vi "Set supply output on first loop.vi"(4 "Current":dbl=300.0 format="%#_gA", 6 "Voltage rise time":dbl=5.0 format="%#_13gs", 7 "Voltage":dbl=52.0 min=0.0 format="%.2fV", 9 "Numeric":i32, 10 "Power supply watchdog time":dbl=2.0 min=0.0 max=10.0 step=0.1 format="%#_13gs", 11 "VISA Refnum in":refnum<visa-resource-name>) -> (0 "error out":errorcluster, 3 "VISA Refnum out":refnum<visa-resource-name>)   [LabVIEW 2024]
uses:
  <userlib>/ZeroJet/IT6000C/IT6000C production.lvlib
  <instrlib>/IT6000C/IT6000C.lvlib
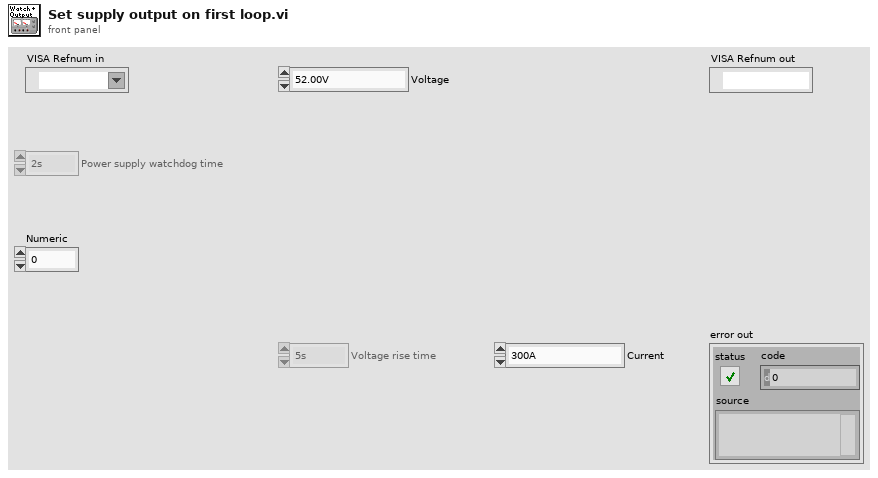
[diagram p1: front panel]
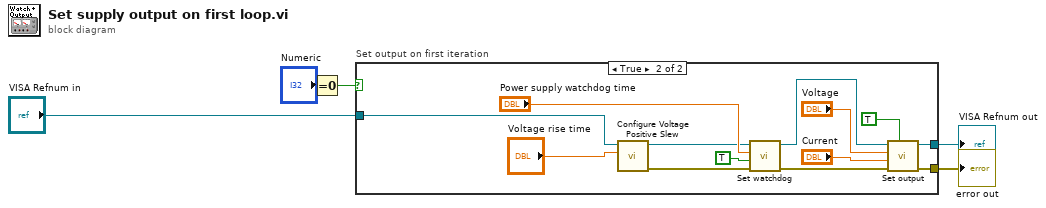
[diagram p0: block diagram]
diagram:
  n1 = Equal To 0?(x="Numeric") -> (x = 0?=w5:bool)
  n2 = case "Set output on first iteration" shown="True" w5 {
    tunnel: "VISA Refnum in" -> [w6 w9]
    tunnel: [w6 w19] -> w1
    tunnel: [_ w17] -> w2
    frame False {
    }
    frame True {
      n3 = call <instrlib>:"Configure Voltage Positive Slew.vi"("Slew"="Voltage rise time", "VISA resource name"=w9) -> ("error out"=w7:errorcluster, "VISA resource name out"=w8:refnum<visa-resource-name>)  [unwired: 8 in]
      n4 = call <userlib>:"Set watchdog.vi"("error in"=w7, "Enable watchdog?"=TRUE, "Time (s)"="Power supply watchdog time", "VISA resource name"=w8) -> ("error out"=w13:errorcluster, "VISA resource name out"=w14:refnum<visa-resource-name>)  [unwired: 6 in]
      n5 = call <userlib>:"Set output.vi"("Output state"=TRUE, "error in"=w13, "Current(A)"="Current", "Voltage(V)"="Voltage", "VISA resource name"=w14) -> ("error out"=w17:errorcluster, "VISA resource name out"=w19:refnum<visa-resource-name>)  [unwired: 5 in]
    }
  }
  "error out" <- w2
  "VISA Refnum out" <- w1
